vi "AGCxxx Reset.vi"(0 "AGCxxx VISA Cluster":T1={"VISA resource name"="", "VISA Timeout Value (1000 ms)"=1000, "Lock Timeout (1000 ms)"=1000, "MAX Channel (6)"=6}, 11 "error in (no error)":errorcluster) -> (4 "dup AGCxxx VISA Cluster":T1={"VISA resource name"="", "VISA Timeout Value (1000 ms)"=1000, "Lock Timeout (1000 ms)"=1000, "MAX Channel (6)"=6}, 15 "error out":errorcluster)   [LabVIEW 2014, in "AGCxxx - Driver.lvlib"]
doc: "This VI resets the instrument, and then sends a set of default setup commands to the instrument. If a Reset command is not supported, it will return a warning.\n\n! THE AGC NEEDS 12 SECONDS TO RESET !\n\nCopyright (C) \nGesellschaft f. Schwerionenforschung, GSI\nPlanckstr. 1\n64291 Darmstadt\nGermany\n\nContact: http://www-wnt.gsi.de/labview\n H.Brand@gsi.de\n\nThis program is free software; you can redistribute it and/or\nmodify it under the terms of the GNU General Public License\nas published by the Free Software Foundation; either version 2\nof the License, or (at your option) any later version.\n\nThis program is distributed in the hope that it will be useful,\nbut WITHOUT ANY WARRANTY; without even the implied warranty of\nMERCHANTABILITY or FITNESS FOR A PARTICULAR PURPOSE. See the\nGNU General Public License for more details (http://www.gnu.org)."
uses:
  AGCxxx - Driver.lvlib
  AGCxxx VISA Control.ctl
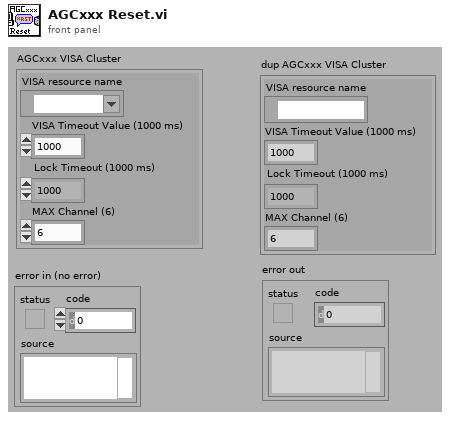
[diagram p1: front panel]
types:
  T1 = typedef "AGCxxx - Driver.lvlib/AGCxxx VISA Control.ctl" = cluster{"VISA resource name":refnum<visa-resource-name>, "VISA Timeout Value (1000 ms)":u32, "Lock Timeout (1000 ms)":u32, "MAX Channel (6)":i32}
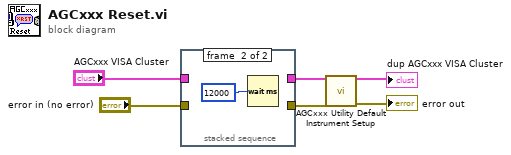
[diagram p0: block diagram]
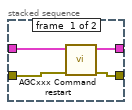
[diagram p2: hidden frame]
diagram:
  n1 = stacked-sequence {
    tunnel: "AGCxxx VISA Cluster" -> [w10 _]
    tunnel: [w9 _] -> w4
    tunnel: [w8 _] -> w3
    tunnel: "error in (no error)" -> [w7 _]
    frame #0 {
      n2 = call "AGCxxx Command restart.vi"("error in (no error)"=w7, "AGCxxx VISA Cluster"=w10) -> ("error out"=w8:errorcluster, "dup AGCxxx VISA Cluster"=w9:T1)  [unwired: 6 in, 1 out]
    }
    frame #1 {
      n3 = Wait (ms)(milliseconds to wait=u32 12000) -> ()  [unwired: 1 out]
    }
  }
  n4 = call "AGCxxx Utility Default Instrument Setup.vi"("AGCxxx VISA Cluster"=w4, "error in (no error)"=w3) -> ("dup AGCxxx VISA Cluster"=→"dup AGCxxx VISA Cluster":T1, "error out"=→"error out":errorcluster)  [unwired: 12 in]
